vi "System Tests.vi"() -> ()   [LabVIEW 2021]
uses:
  Source/Support/Nodes/abs_Node/Status.ctl
  Source/System/bt_System.lvclass
  Source/Support/Nodes/Decorators/Repeater/Support/Finish On - Type.ctl
  Source/System/bt_System.lvclass/bt_System.ctl
  Source/System/Properties/Write Behaviour Tree.vi
  Source/BT.lvlib
  Source/Support/Nodes/Decorators/Repeater/bt_Repeater.lvclass
  Source/Support/Nodes/abs_Node/bt_Node.lvclass
panel:
  in  "stop":bool
  out "Status 2":T1
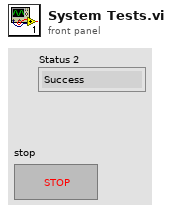
[diagram p1: front panel]
types:
  T1 = typedef "BT.lvlib/bt_Node.lvclass/Status.ctl" = enum16{"Success", "Failure", "Running"}
  T2 = typedef "BT.lvlib/bt_Repeater.lvclass/Finish On - Type.ctl" = enum16{"Success", "Failure", "Never"}
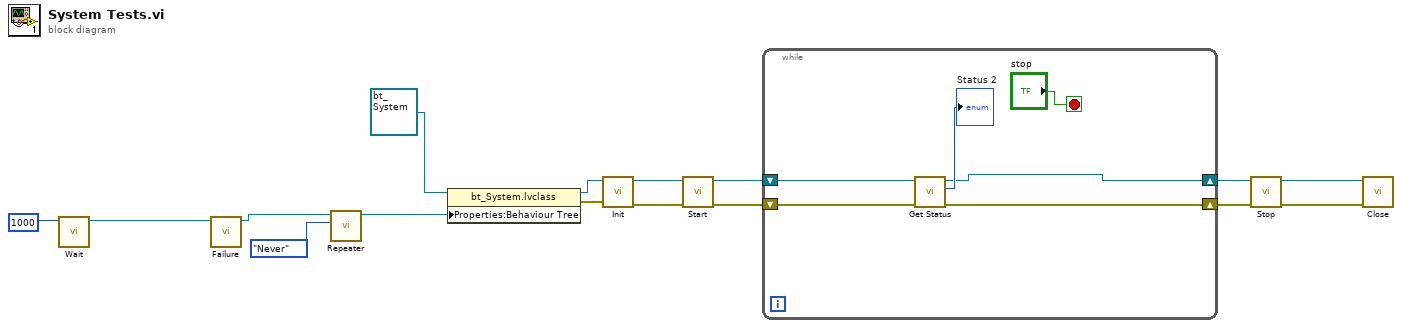
[diagram p0: block diagram]
diagram:
  n1 = call "Wait.vi"("Time (ms)"=u32 1000) -> ("Node Out"=w5:refnum<class "bt_Node.lvclass">)  [unwired: 10 in]
  n2 = call "Failure.vi"("Node In"=w5) -> ("Node"=w10:refnum<class "bt_Node.lvclass">)  [unwired: 10 in]
  n3 = call "Repeater.vi"("Finish On"=Finish_On_-_Type."Never", "Node In"=w10) -> ("Node Out"=w13:refnum<class "bt_Node.lvclass">)  [unwired: 9 in]
  n4 = property class="bt_System.lvclass"(reference=refnum<class "bt_System.lvclass"> refnum ("bt_System in"), "Properties:Behaviour Tree"=w13) -> (reference out=w14:refnum<class "bt_System.lvclass">, error out=w16:errorcluster)  [unwired: 1 in]
  n5 = call "Init.vi"("error in (no error)"=w16, "bt_System in"=w14) -> ("error out"=w4:errorcluster, "bt_System out"=w3:refnum<class "bt_System.lvclass">)  [unwired: 8 in]
  n6 = call "Start.vi"("error in (no error)"=w4, "bt_System in"=w3) -> ("error out"=w2:errorcluster, "bt_System out"=w1:refnum<class "bt_System.lvclass">)  [unwired: 8 in]
  n7 = while {
    shift-right: [w18] -> w8
    shift-left: w1 -> [w22]
    shift-right: [w19] -> w9
    shift-left: w2 -> [w21]
    stop <- "stop" stop-if-true
    n8 = call "Get Status.vi"("error in (no error)"=w21, "bt_System in"=w22) -> ("error out"=w19:errorcluster, "Status"=→"Status 2":T1, "bt_System out"=w18:refnum<class "bt_System.lvclass">)  [unwired: 7 in]
  }
  n9 = call "Stop.vi"("error in (no error)"=w9, "bt_System in"=w8) -> ("error out"=w6:errorcluster, "bt_System out"=w7:refnum<class "bt_System.lvclass">)  [unwired: 8 in]
  n10 = call-dynamic "Close.vi"("error in (no error)"=w6, "bt_System in"=w7) -> ()  [unwired: 8 in, 2 out]
